vi "Util.Error.Build.vi"(6 "Suppress call-chain info.":bool, 8 "error in (no error)":errorcluster, 9 "Status":bool=TRUE, 10 "code":i32=-1, 11 "Source":string) -> (0 "error out":errorcluster)   [LabVIEW 2020]
panel:
  # "Util.Error.Build.vi\n\nAppends new detail to existing error-detail.\n\nPlease visit http://www.OpenG.org to learn about the\nOpen Source LabVIEW software movement.\n\nNOTICE -- YOU MUST LEAVE THIS NOTICE IN PLACE.  PER THE TERMS OF THE LICENSE BELOW, YOU MAY SUBLICENSE THIS SOFTWARE \nIN ANY WAY THAT DOES NOT CONFLICT WITH THIS LICENSE.\n\n### BSD License (http://www.opensource.org/licenses/bsd-license.php) Begin ###\n \nCopyright (c) 2007, Bill Clench <bclench@yahoo.com>\n\nAll rights reserved.\n\nRedistribution and use in source and binary forms, with or without modification, are permitted provided that the following conditions are met:\n\n    * Redistributions of source code must retain the above copyright notice, this list of conditions and the following disclaimer.\n    * Redistributions in binary form must reproduce the above copyright notice, this list of conditions and the following disclaimer in the \n       documentation and/or other materials provided with the distribution.\n    * Neither the name of SciWare, James Kring, Inc., nor the names of its contributors may be used to endorse or promote products derived \n       from this software without specific prior written permission.\n\nTHIS SOFTWARE IS PROVIDED BY THE COPYRIGHT HOLDERS AND CONTRIBUTORS \"AS IS\" AND ANY EXPRESS OR IMPLIED WARRANTIES, \nINCLUDING, BUT NOT LIMITED TO, THE IMPLIED WARRANTIES OF MERCHANTABILITY AND FITNESS FOR A PARTICULAR PURPOSE ARE \nDISCLAIMED. IN NO EVENT SHALL THE COPYRIGHT OWNER OR CONTRIBUTORS BE LIABLE FOR ANY DIRECT, INDIRECT, INCIDENTAL,\n SPECIAL, EXEMPLARY, OR CONSEQUENTIAL DAMAGES (INCLUDING, BUT NOT LIMITED TO, PROCUREMENT OF SUBSTITUTE GOODS OR \nSERVICES; LOSS OF USE, DATA, OR PROFITS; OR BUSINESS INTERRUPTION) HOWEVER CAUSED AND ON ANY THEORY OF LIABILITY, \nWHETHER IN CONTRACT, STRICT LIABILITY, OR TORT (INCLUDING NEGLIGENCE OR OTHERWISE) ARISING IN ANY WAY OUT OF THE USE \nOF THIS SOFTWARE, EVEN IF ADVISED OF THE POSSIBILITY OF SUCH DAMAGE.\n\n### BSD License End ###"
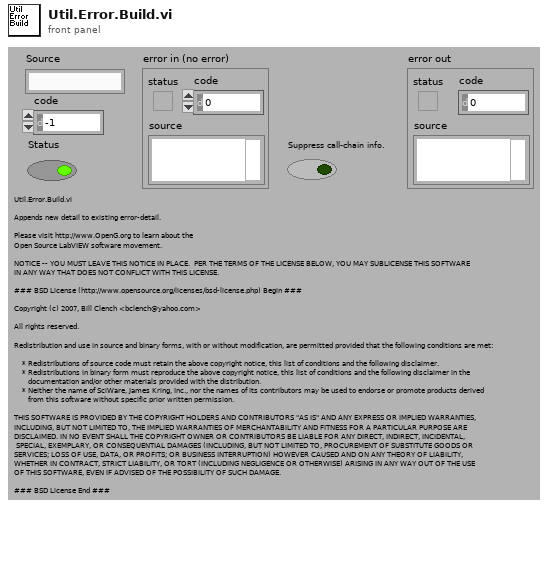
[diagram p1: front panel]
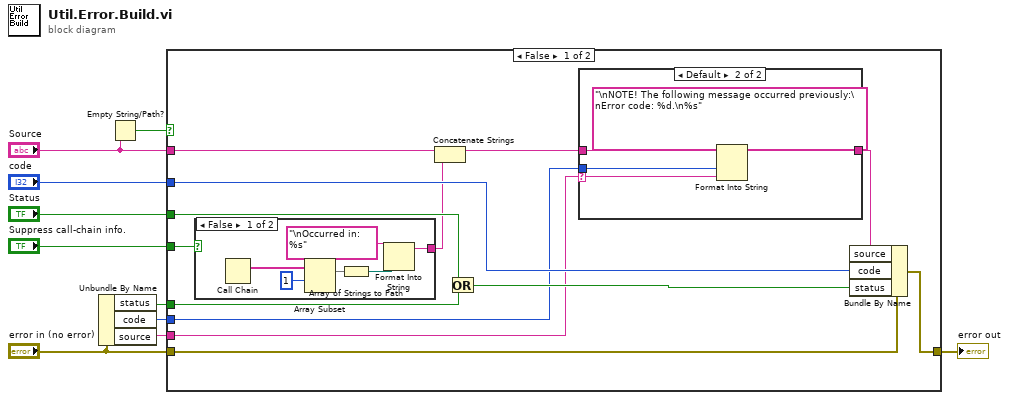
[diagram p0: block diagram]
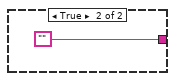
[diagram p2: hidden frame]
diagram:
  n1 = Unbundle By Name("error in (no error)") -> ("status"=w9:bool, "code"=w1:i32, "source"=w5:string)
  n2 = Empty String/Path?(string/path="Source") -> (empty?=w3:bool)
  n3 = case shown="False" w3 {
    tunnel: "Status" -> [w23 _]
    tunnel: w9 -> [w22 _]
    tunnel: "error in (no error)" -> [w21 w37]
    tunnel: [w19 w37] -> w7
    tunnel: "code" -> [w18 _]
    tunnel: w5 -> [w16 _]
    tunnel: "Source" -> [w15 _]
    tunnel: "Suppress call-chain info." -> [w12 _]
    tunnel: w1 -> [w11 _]
    frame False {
      n4 = case shown="False" w12 {
        tunnel: [w28 ""] -> w14
        frame False {
          n5 = Call Chain() -> (call chain=w26:string[])
          n6 = Array Subset(array=w26, index=1) -> (w27:string[])  [unwired: 1 in]
          n7 = Array of Strings to Path(0:w27) -> (2:w24:path)  [unwired: 1 in]
          n8 = Format Into String(format string="\nOccurred in: %s", w24) -> (resulting string=w28:string)  [unwired: 2 in, 1 out]
        }
        frame True {
        }
      }
      n9 = Concatenate Strings(w15, w14) -> (w13:string)
      n10 = Or(x=w23, y=w22) -> (x .or. y?=w20:bool)
      n11 = case shown="Default" w16 {
        selector: w16 -> [_ w33]
        tunnel: [w31 w35] -> w17
        tunnel: w13 -> [w31 w34]
        tunnel: w11 -> [_ w32]
        frame "" {
        }
        frame Default {
          n12 = Format Into String(format string="\nNOTE! The following message occurred previously:\nError code: %d.\n%s", initial string=w34, w32, w33) -> (resulting string=w35:string)  [unwired: 1 in, 1 out]
        }
      }
      n13 = Bundle By Name(cluster=w21, "source"=w17, "code"=w18, "status"=w20) -> (w19:errorcluster)
    }
    frame True {
    }
  }
  "error out" <- w7
